vi "GF_WaypointGoodness.vi"() -> ()   [LabVIEW 2012]
panel:
  out "GF_WaypointGoodness":dbl
  in  "Heading to Waypoint":dbl
  in  "Test Heading":dbl
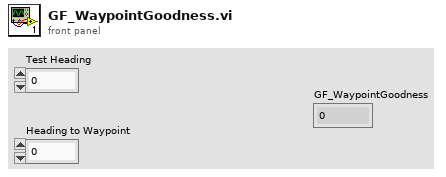
[diagram p1: front panel]
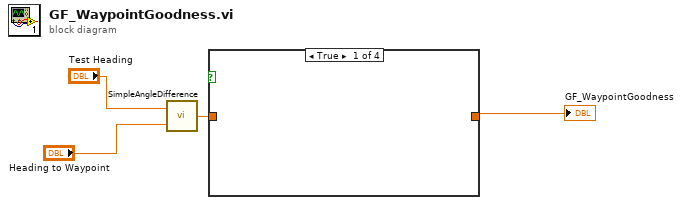
[diagram p0: block diagram]
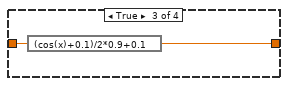
[diagram p3: hidden frame]
diagram:
  n1 = call "SimpleAngleDifference.vi"("Angle 2"="Heading to Waypoint", "Angle 1"="Test Heading") -> ("Difference"=w2:dbl)
  n2 = case shown="\"Wide\"" {
    selector: _ -> [_ _ _ _]
    tunnel: w2 -> [_ _ w6 _]
    tunnel: [_ _ w5 _] -> w1
    frame True {
    }
    frame False {
    }
    frame True {
      n3 = expression code="(cos(x)+0.1)/2*0.9+0.1"(w6) -> (w5:dbl)
    }
    frame True {
    }
  }
  "GF_WaypointGoodness" <- w1
